vi "Main.vi"(8 "error in":errorcluster) -> (0 "error out":errorcluster)   [LabVIEW 2021, in "Interface-Module.lvlib"]
doc: "This template is based from the Queued Message Handler design pattern and the Queued Message Handler Project Template that ships with LabVIEW 2014.\n\nThe main difference is that the Queue is private to this module and communication between modules is done via Broadcast and Request events.\n\nRequest events are wrapped via public API methods and are handled in the Event handler loop in this VI.\nAny module can register for Broadcast events sent by this module.\n\nThe Event Handling Loop generates messages based on user interface actions.\n\nThe Message Handling Loop processes messages generated by the Event Handling Loop, or by other messages. The messages are string values, so new messages can be added easily to the Message Cases case structure in the Message Handling Loop. Each message cluster can also provide an optional value for Message Data, which is a variant that can be converted to whatever message-specific data is required.\n_____\nBased on Delacor QMH Project Template 3.0.0.32."
uses:
  Interface-Module.lvlib
  <vilib>/Delacor/Delacor QMH/Libraries/Module Admin_class/Delacor_lib_QMH_Module Admin.lvclass
  Module Data--cluster.ctl
  <vilib>/Delacor/Delacor QMH/Libraries/Message Queue_class/Delacor_lib_QMH_Message Queue.lvclass/Delacor_lib_QMH_Message Queue.ctl
  Valve-Module/Module/Controls/valve-cmd.ctl
  Show Panel Argument--cluster.ctl
  Hide Panel Argument--cluster.ctl
  Stop Argument--cluster.ctl
  <vilib>/Delacor/Delacor QMH/Libraries/Module Admin_class/Delacor_lib_QMH_Module Admin.lvclass/Delacor_lib_QMH_Module Admin.ctl
  <vilib>/Utility/miscctls.llb/LVPointTypeDef.ctl
  <vilib>/Delacor/Delacor QMH/Libraries/Message Queue_class/Delacor_lib_QMH_Enqueue Message (Single).vi
  <vilib>/Delacor/Delacor QMH/Libraries/Module Admin_class/Delacor_lib_QMH_Get External Launch.vi
  <vilib>/Utility/error.llb/Error Cluster From Error Code.vi
  <vilib>/ErrorRing/Error Ring.xnode
  <vilib>/Delacor/Delacor QMH/Libraries/Message Queue_class/Delacor_lib_QMH_Message Queue.lvclass
  Temperature-Module/Temperature-Module.lvlib
  Valve-Module/Valve-Module.lvlib
  Pressure Module/Pressure Module.lvlib
  Actuator Module/Actuator Module.lvlib
panel:
  out "Flow  2":dbl format="%_3g"
  out "Flow  1":dbl format="%_3g"
  out "P 5":dbl format="%_3g"
  out "P 4":dbl format="%_3g"
  out "P 3":dbl format="%_3g"
  out "P 2":dbl format="%_3g"
  out "P 1":dbl format="%_3g"
  out "Actuator Read":dbl(slide) scale=0.0..100.0
  out "Valve":bool[](array[boolean])
  out "Temperature":dbl[](array[numeric]) format="%#_4g"
  in  "Actuator\n Control":dbl(slide) scale=0.0..100.0
  in  "Start Display":bool
  in  "Valve 3":bool
  in  "Valve 2":bool
  in  "Valve 1":bool
  in  "Simulate MHL Error":bool
  in  "Simulate EHL Error":bool
  in  "Module Admin":refnum<class "Delacor_lib_QMH_Module Admin.lvclass">
  out "Status":string
  # "Distillation Column"
  # "Display"
  # "Control"
  # "Flow Meter"
  # "%"
  # "Pressure"
  # "Valve 1"
  # "Valve 2"
  # "Valve 3"
  # "Top"
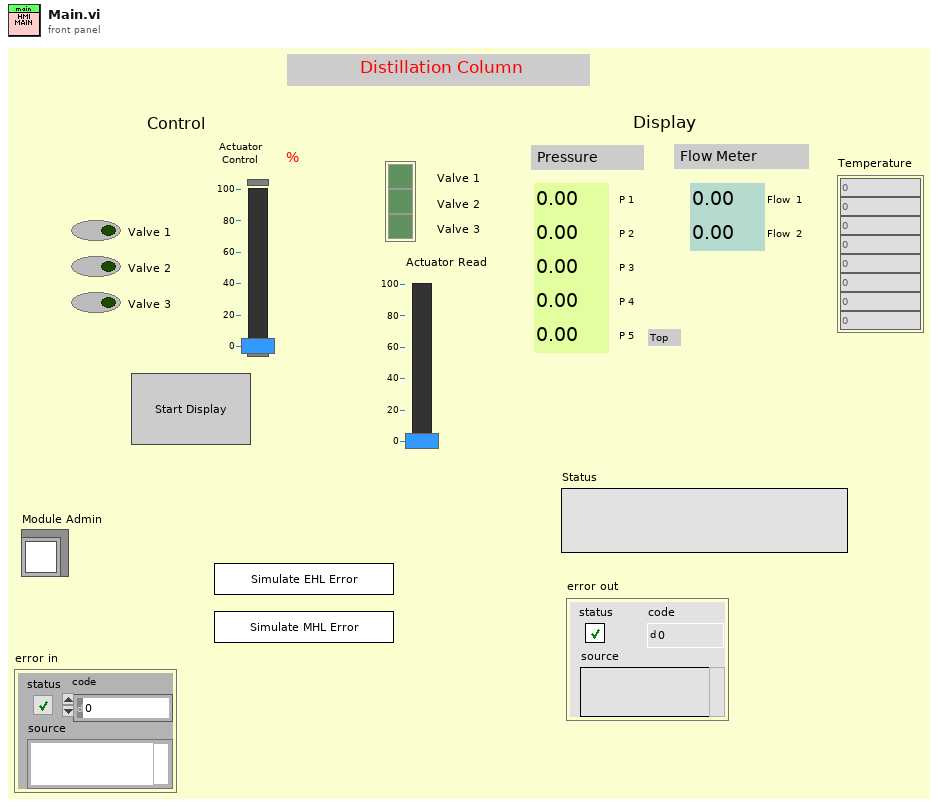
[diagram p1: front panel]
types:
  T1 = typedef "Interface-Module.lvlib/Request Events--cluster.ctl" = cluster{"Stop Module":refnum<user-event>, "Show Panel":refnum<user-event>, "Hide Panel":refnum<user-event>, "Get Module Execution Status":refnum<user-event>, "Show Diagram":refnum<user-event>}
  T2 = typedef "Temperature-Module.lvlib/Broadcast Events--cluster.ctl" = cluster{"Status Updated":refnum<user-event>, "Send Temperature to HMI":refnum<user-event>}
  T3 = typedef "Valve-Module.lvlib/Broadcast Events--cluster.ctl" = cluster{"Status Updated":refnum<user-event>, "Send-valve-interface":refnum<user-event>}
  T4 = typedef "Pressure Module.lvlib/Broadcast Events--cluster.ctl" = cluster{"Status Updated":refnum<user-event>, "Write pressure to HMI":refnum<user-event>}
  T5 = typedef "Actuator Module.lvlib/Broadcast Events--cluster.ctl" = cluster{"Status Updated":refnum<user-event>, "Actuator-display-Interface":refnum<user-event>}
  T6 = typedef "Interface-Module.lvlib/Module Data--cluster.ctl" = cluster{"Status":string}
  T7 = typedef "valve-cmd.ctl" = cluster{"Valve":bool, "Vavle Seq":i32}
  T8 = typedef "Interface-Module.lvlib/Show Panel Argument--cluster.ctl" = cluster{"Show Panel?":bool}
  T9 = typedef "Interface-Module.lvlib/Hide Panel Argument--cluster.ctl" = cluster{"Hide Panel?":bool}
  T10 = typedef "Interface-Module.lvlib/Stop Argument--cluster.ctl" = cluster{"Origin":string, "Exit via Stop Module Req?":bool, "Wait for Module to stop?":bool}
  T11 = typedef "LVPointTypeDef.ctl" = cluster{"Horizontal":i16, "Vertical":i16}
  T12 = enum32{"Invalid", "Standard", "Closed", "Hidden", "Minimized", "Maximized"}
  T13 = enum32{"invalid lock state", "Not Locked", "Locked (No Password)", "Password-protected"}
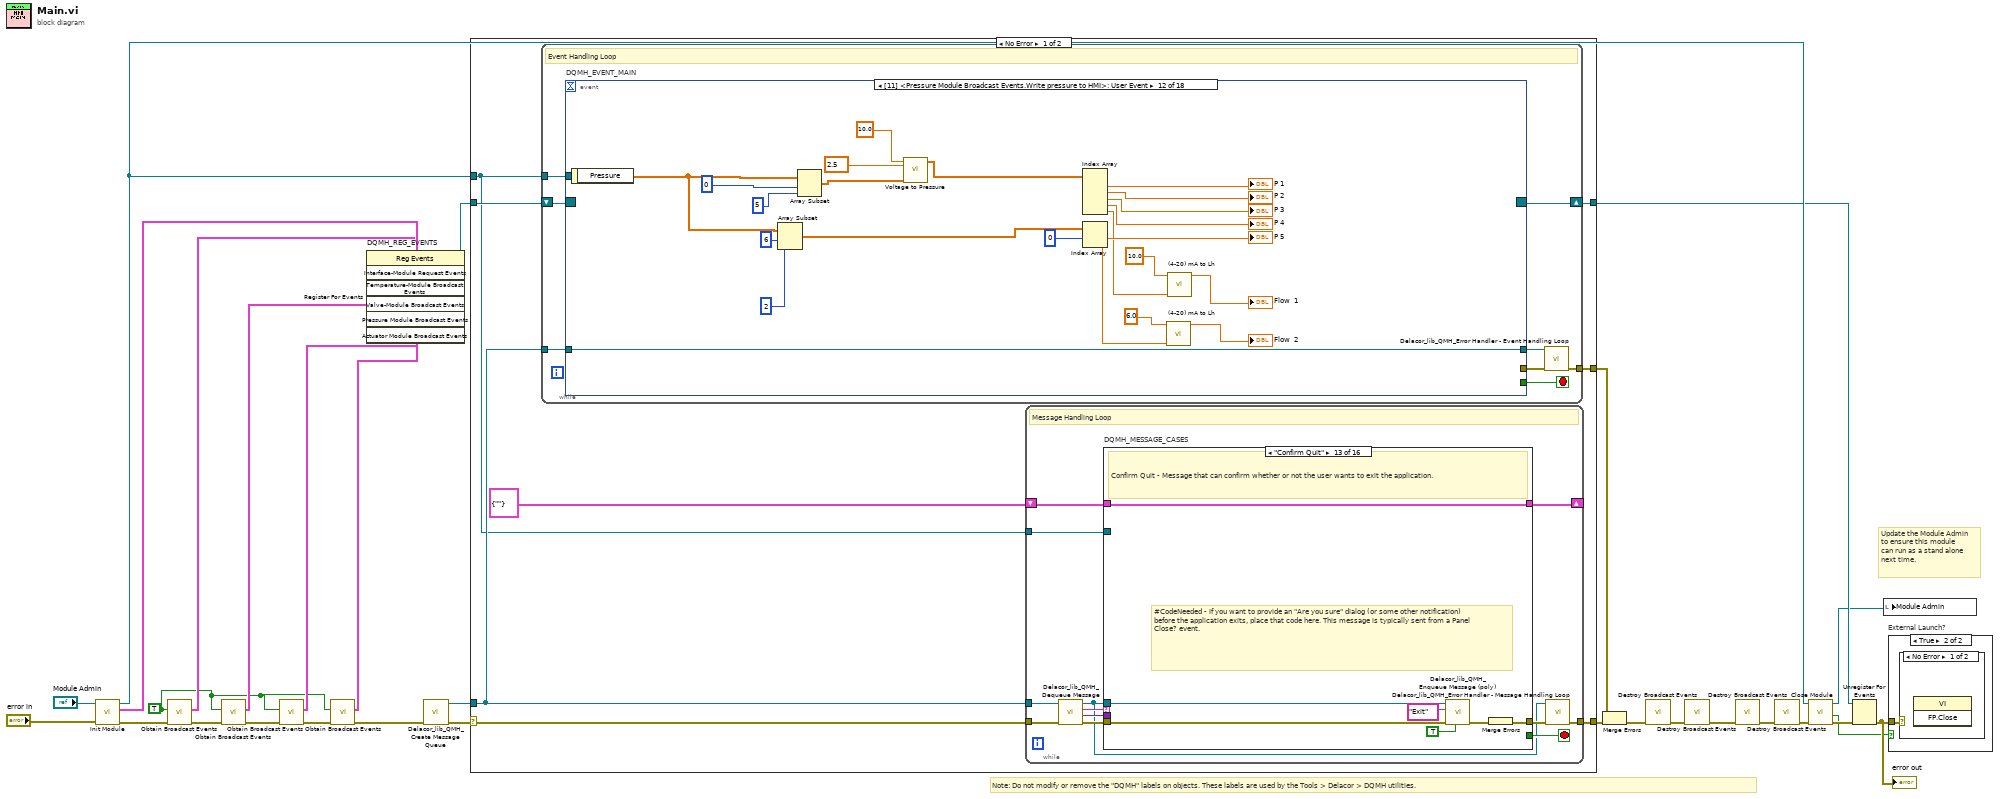
[diagram p0: block diagram]
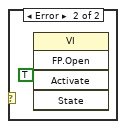
[diagram p3: hidden frame]
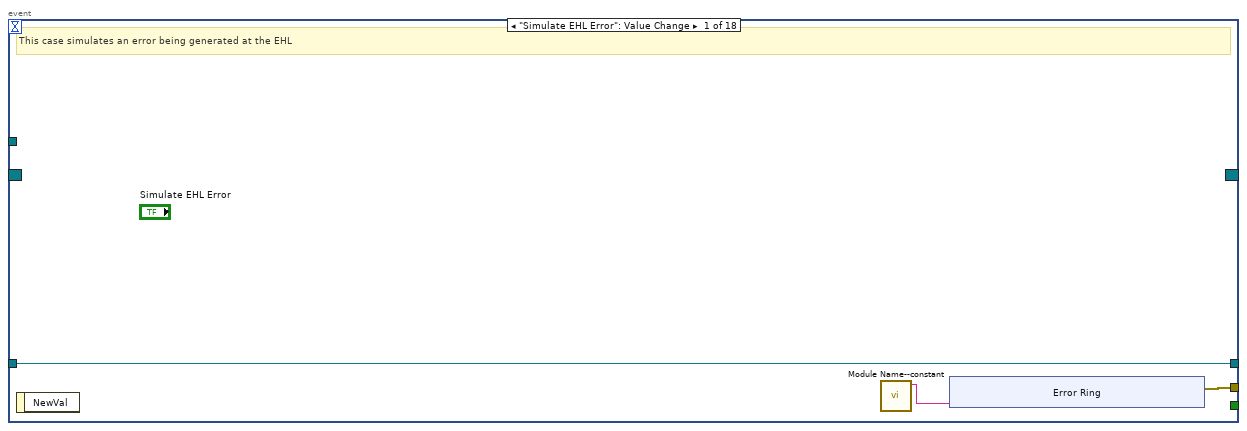
[diagram p4: hidden frame]
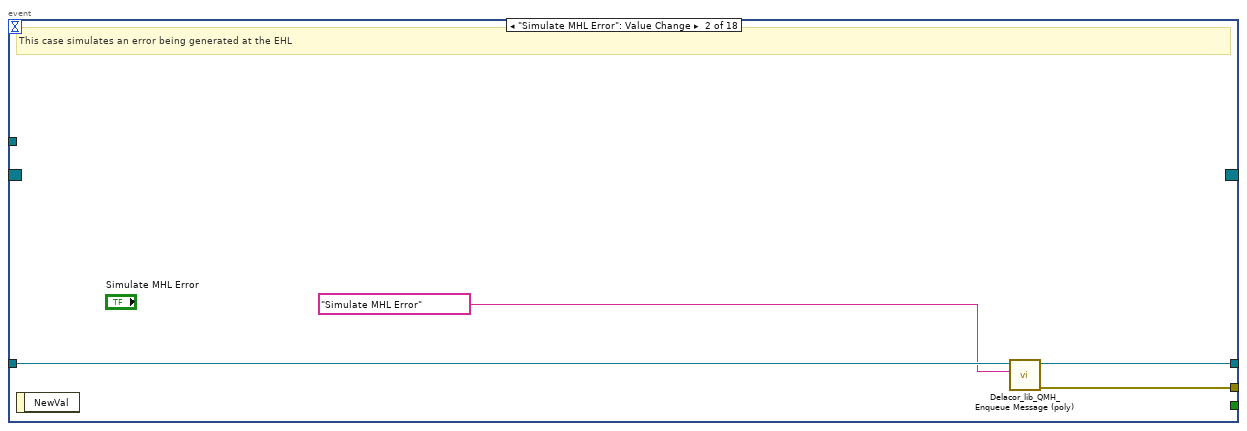
[diagram p5: hidden frame]
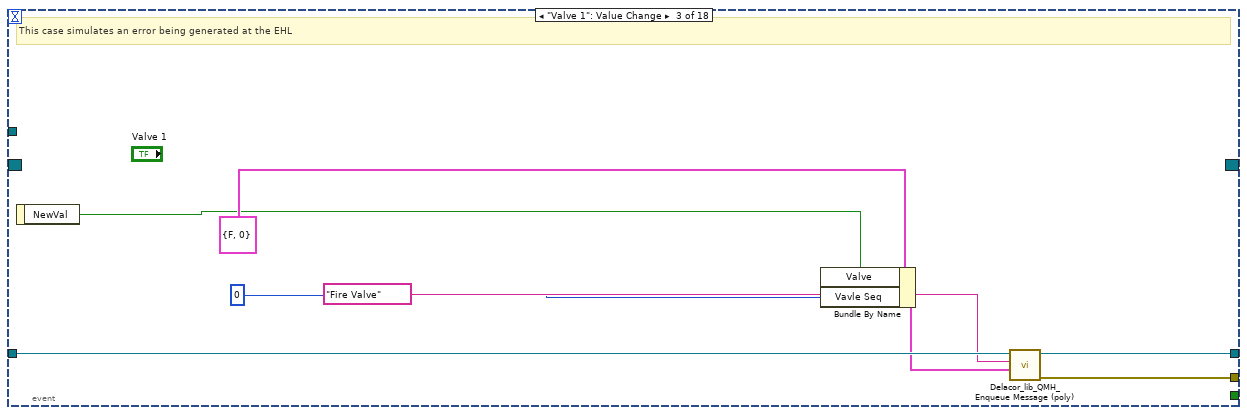
[diagram p6: hidden frame]
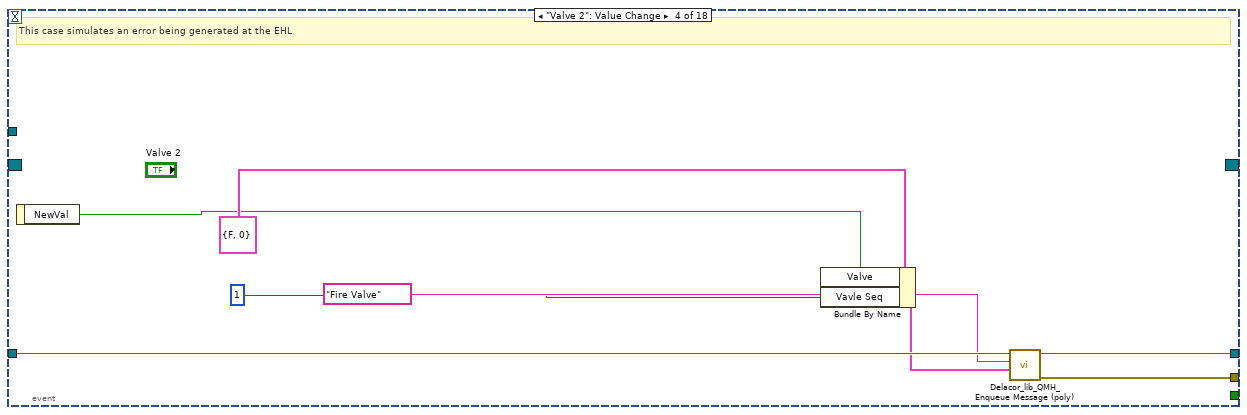
[diagram p7: hidden frame]
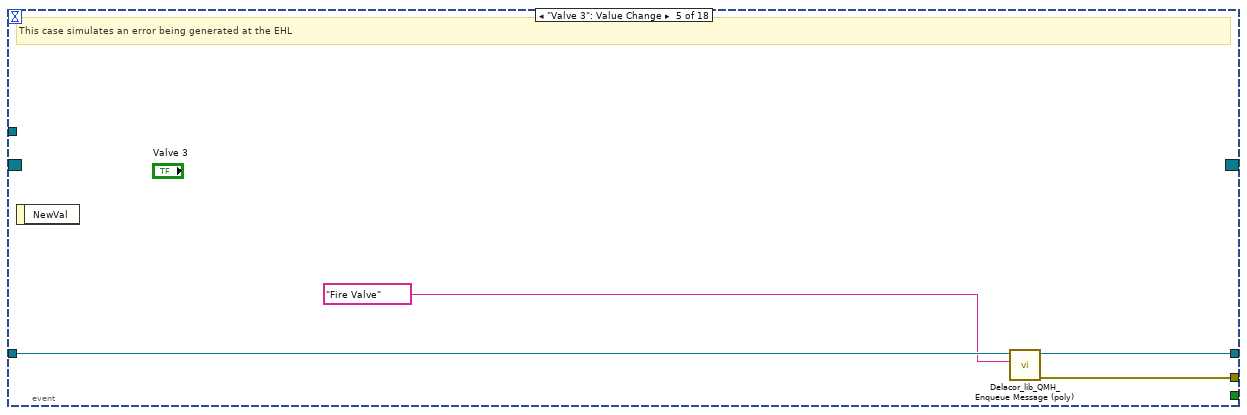
[diagram p8: hidden frame]
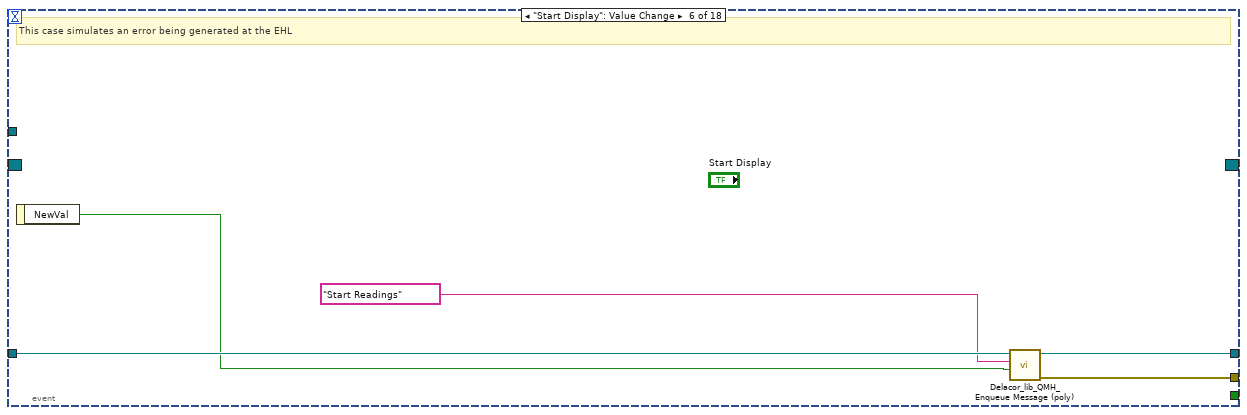
[diagram p9: hidden frame]
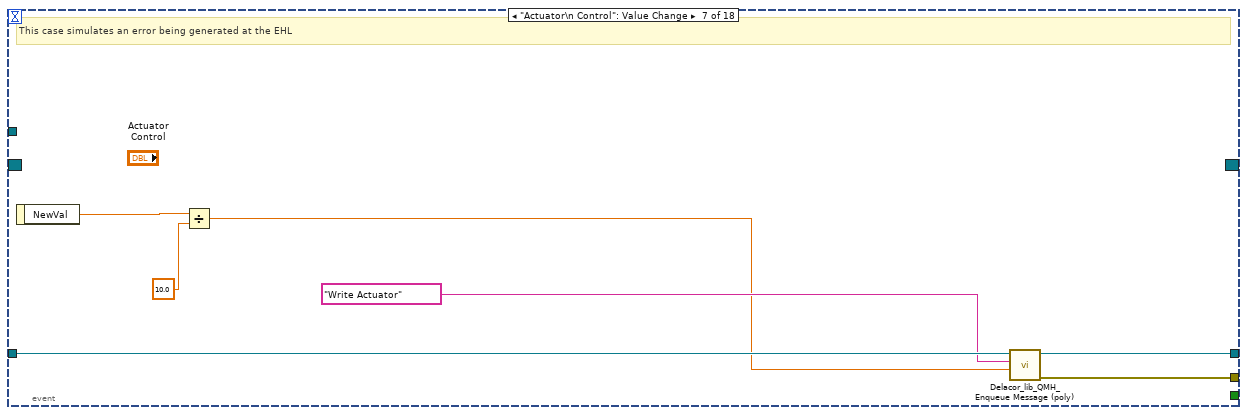
[diagram p10: hidden frame]
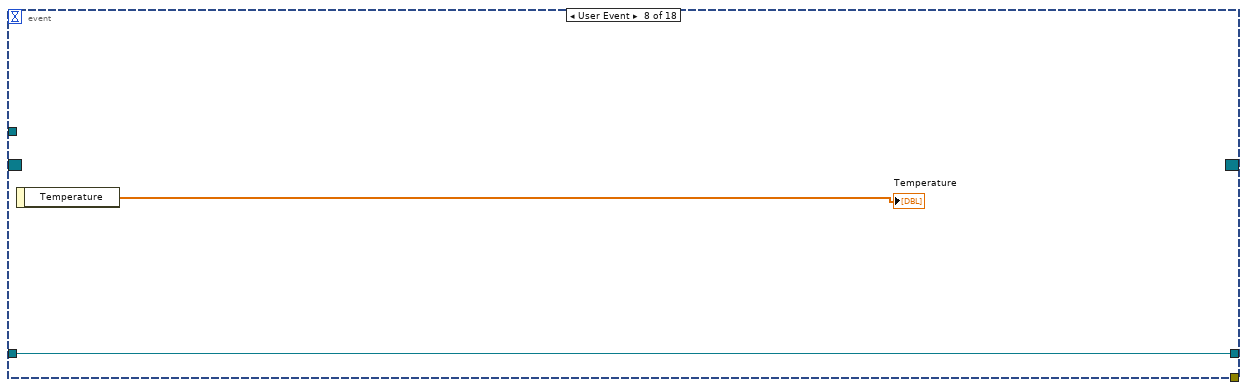
[diagram p11: hidden frame]
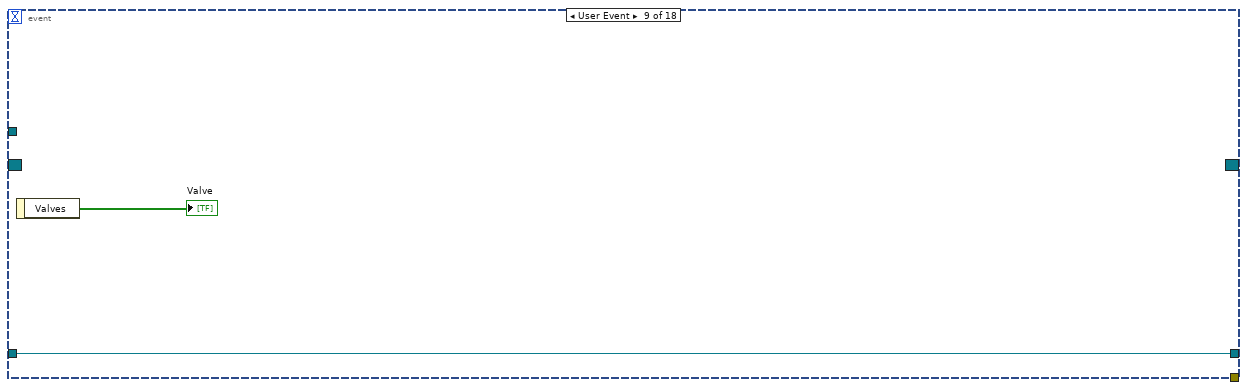
[diagram p12: hidden frame]
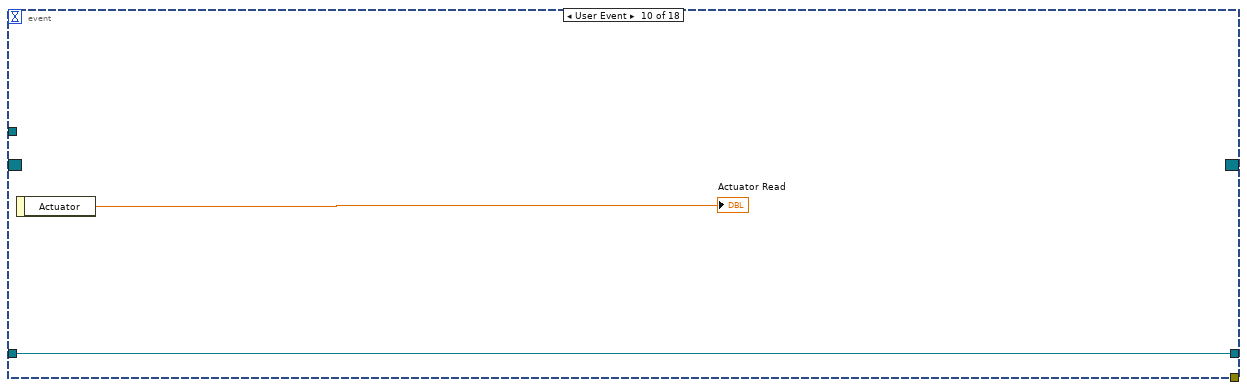
[diagram p13: hidden frame]
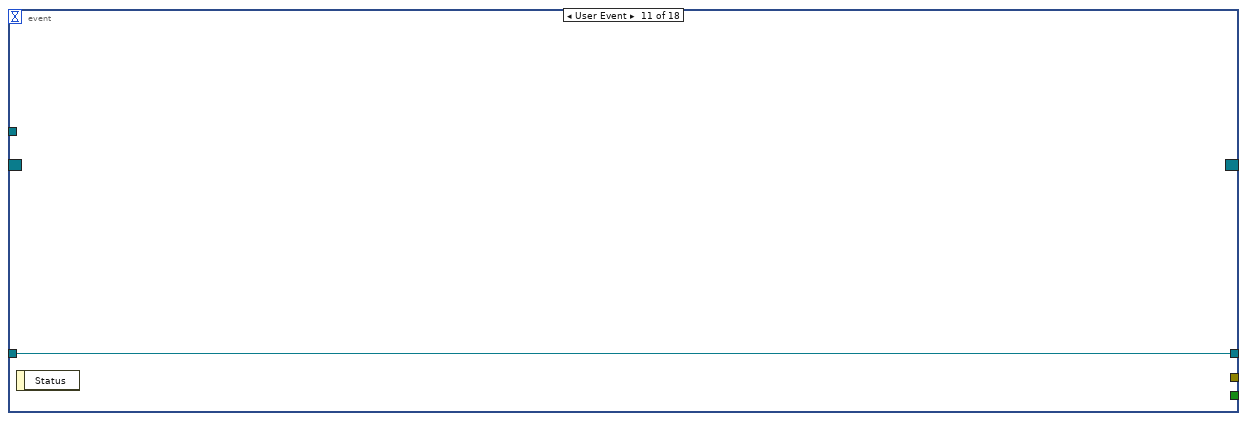
[diagram p14: hidden frame]
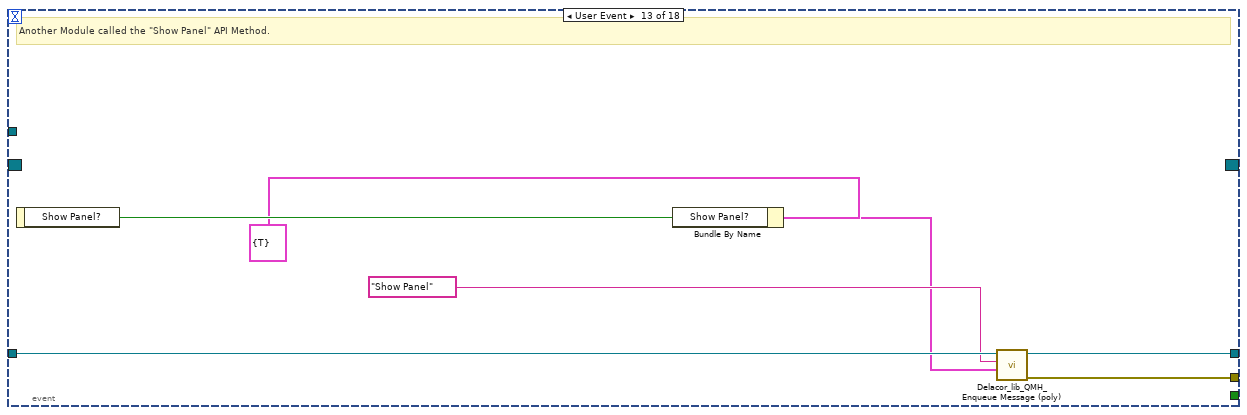
[diagram p15: hidden frame]
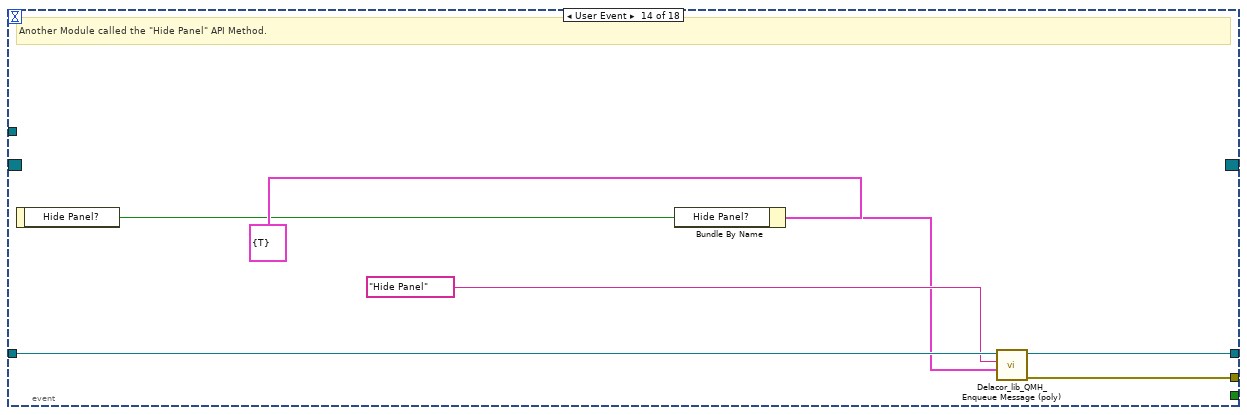
[diagram p16: hidden frame]
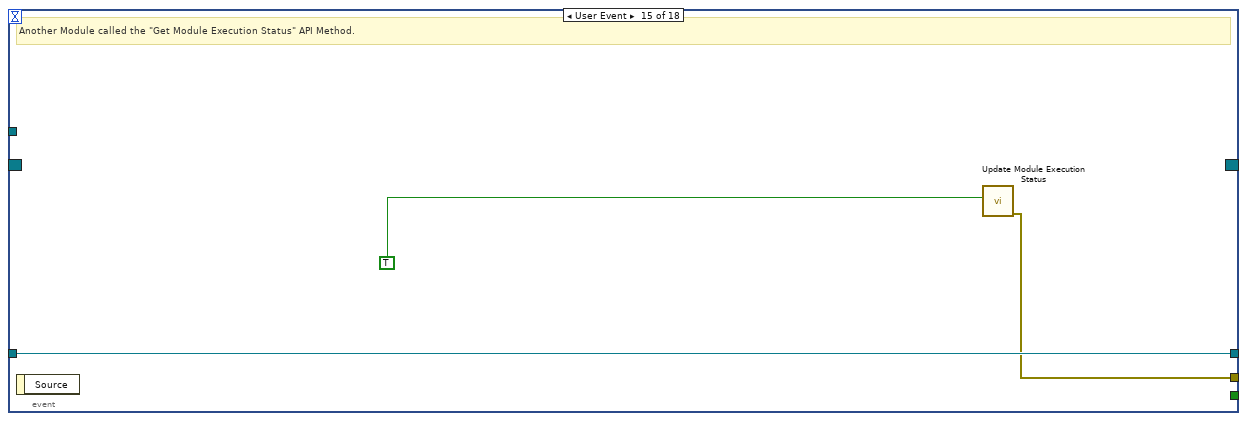
[diagram p17: hidden frame]
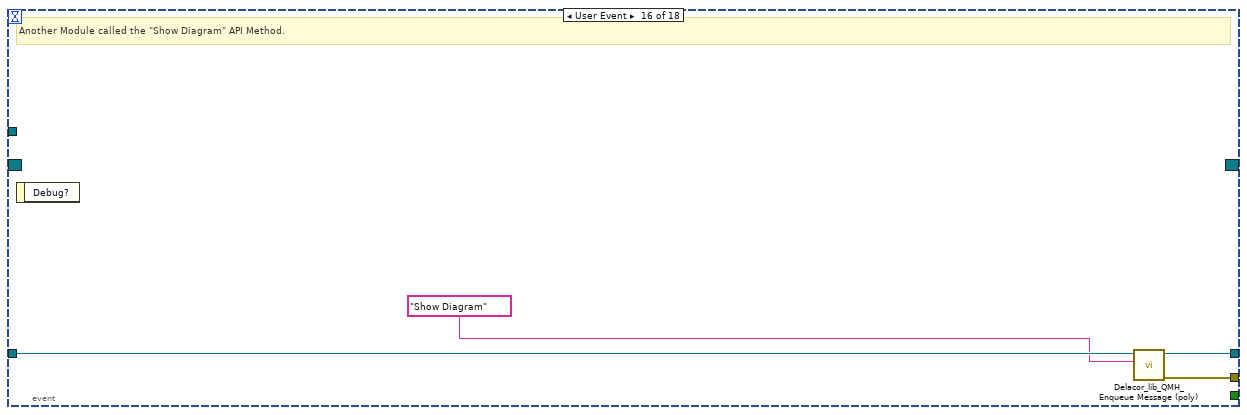
[diagram p18: hidden frame]
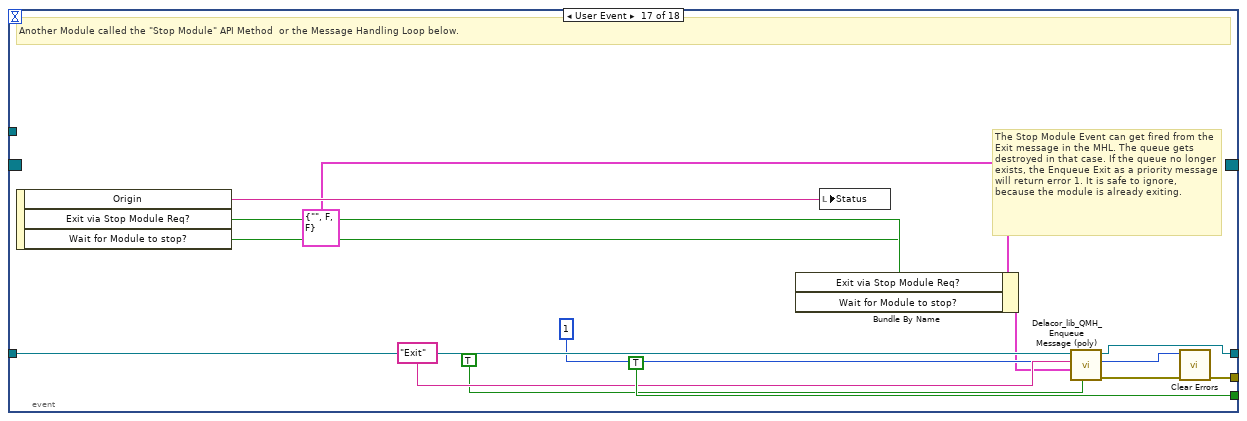
[diagram p19: hidden frame]
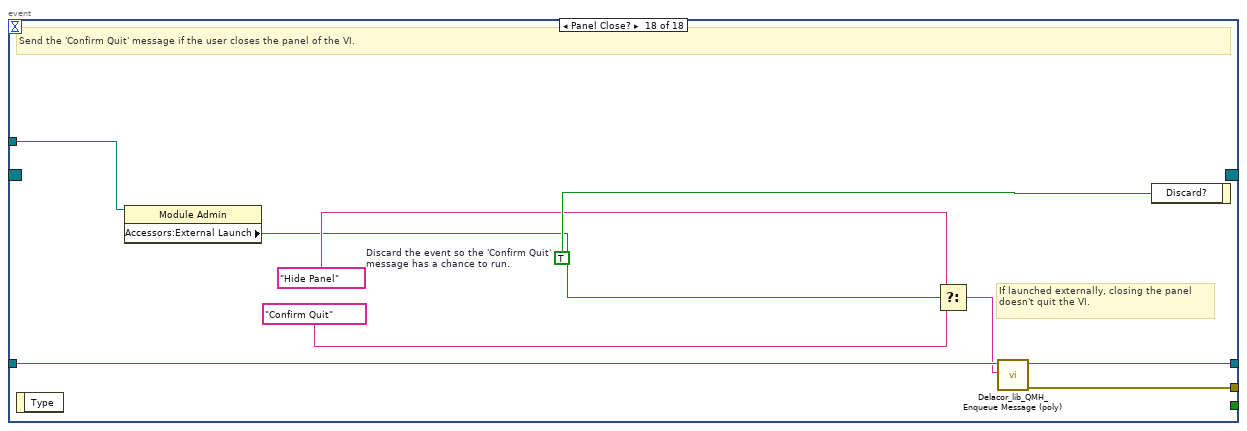
[diagram p20: hidden frame]
diagram:
  w4 = TRUE ("Create New?")
  # "Note: Do not modify or remove the \"DQMH\" labels on objects. These labels are used by the Tools > Delacor > DQMH utilities."
  # "Update the Module Admin to ensure this module can run as a stand alone next time."
  n1 = call "Init Module.vi"("error in (no error)"="error in", "Singleton Module Admin in"="Module Admin") -> ("error out"=w16:errorcluster, "Interface-Module Request Events"=w25:T1, "Singleton Module Admin out"=w29:refnum<class "Delacor_lib_QMH_Module Admin.lvclass">)  [unwired: 7 in]
  n2 = call "Obtain Broadcast Events.vi"("error in (no error)"=w16, "Create New?"=w4) -> ("error out"=w13:errorcluster, "Temperature-Module Broadcast Events"=w15:T2)  [unwired: 8 in]
  n3 = call "Obtain Broadcast Events.vi"("error in (no error)"=w13, "Create New?"=w4) -> ("error out"=w10:errorcluster, "Valve-Module Broadcast Events"=w12:T3)  [unwired: 8 in]
  n4 = call "Obtain Broadcast Events.vi"("error in (no error)"=w10, "Create New?"=w4) -> ("error out"=w6:errorcluster, "Pressure Module Broadcast Events"=w9:T4)  [unwired: 8 in]
  n5 = call "Obtain Broadcast Events.vi"("error in (no error)"=w6, "Create New?"=w4) -> ("error out"=w5:errorcluster, "Actuator Module Broadcast Events"=w3:T5)  [unwired: 8 in]
  n6 = register-events "DQMH_REG_EVENTS"(w25, w15, w12, w9, w3) -> (reference out=w26:refnum<event-registration>)  [unwired: 2 in, 1 out]
  n7 = call <vilib>:"Delacor_lib_QMH_Create Message Queue.vi"("error in"=w5) -> ("error out"=w17:errorcluster, "Message Queue"=w24:refnum<class "Delacor_lib_QMH_Message Queue.lvclass">)  [unwired: 9 in]
  n8 = case shown="No Error" w17 {
    selector: w17 -> [w31 w331]
    tunnel: [w37 w331] -> w28
    tunnel: [w36 w336] -> w27
    tunnel: w26 -> [w34 w336]
    tunnel: w24 -> [w33 _]
    tunnel: [w32 _] -> w20
    tunnel: w29 -> [w30 w332]
    frame No Error {
      n9 = while {
        tunnel: w33 -> [w45]
        shift-right: [w43] -> w36
        shift-left: w34 -> [w44]
        tunnel: [w39] -> w32
        tunnel: w30 -> [w38]
        stop <- w41 stop-if-true
        # "Event Handling Loop"
        n10 = event "DQMH_EVENT_MAIN" shown="[11] <Pressure Module Broadcast Events.Write pressure to HMI>: User Event" {
          selector: w44 -> [_ _ _ _ _ _ _ _ _ _ _ _ _ _ _ _ _ _]
          dyn-events: [_ _ _ _ _ _ _ _ _ _ _ _ _ _ _ _ _ _] -> w43
          timeout: _ -> [_ _ _ _ _ _ _ _ _ _ _ _ _ _ _ _ _ _]
          tunnel: [_ _ _ _ _ _ _ _ _ _ _ _ _ _ _ _ TRUE ("Discard?") _] -> w41
          tunnel: w45 -> [w48 w59 w67 w75 w79 w84 w91 w93 w95 w97 w98 w121 w128 w135 w138 w142 w153 w163]
          tunnel: [w47 w56 w64 w72 w76 w81 w88 _ _ _ _ _ w126 w133 w137 w139 w147 w162] -> w42
          tunnel: [w48 w58 w66 w74 w78 w83 w90 w93 w95 w97 w98 w121 w127 w134 w138 w141 w152 w161] -> w40
          tunnel: w38 -> [_ _ _ _ _ _ _ _ _ _ _ _ _ _ _ _ _ w157]
          event "Simulate EHL Error": Value Change {
            # "This case simulates an error being generated at the EHL"
            n11 = event-data() -> ()  [unwired: 1 in, 1 out]
            n12 = call "Module Name--constant.vi"() -> ("Module Name"=w46:string)  [unwired: 11 in]
            n13 = xnode "Error Ring"("parameter 0"=w46) -> ("error out"=w47:errorcluster)
          }
          event "Simulate MHL Error": Value Change {
            # "This case simulates an error being generated at the EHL"
            n14 = event-data() -> ()  [unwired: 1 in, 1 out]
            n15 = call-poly <vilib>:"Delacor_lib_QMH_Enqueue Message (poly).vi"("Message"="Simulate MHL Error", "Message Queue in"=w59) -> ("error out"=w56:errorcluster, "Message Queue out"=w58:refnum<class "Delacor_lib_QMH_Message Queue.lvclass">)  [unwired: 8 in]
          }
          event "Valve 1": Value Change {
            # "This case simulates an error being generated at the EHL"
            n16 = event-data() -> ("NewVal"=w62:bool)  [unwired: 1 in]
            n17 = Bundle By Name(cluster=T7 {"Valve"=FALSE, "Vavle Seq"=0} ("Cmd"), "Valve"=w62, "Vavle Seq"=0) -> (w60:T7)
            n18 = call-poly <vilib>:"Delacor_lib_QMH_Enqueue Message (poly).vi"("Message Data"=w60, "Message"="Fire Valve", "Message Queue in"=w67) -> ("error out"=w64:errorcluster, "Message Queue out"=w66:refnum<class "Delacor_lib_QMH_Message Queue.lvclass">)  [unwired: 7 in]
          }
          event "Valve 2": Value Change {
            # "This case simulates an error being generated at the EHL"
            n19 = event-data() -> ("NewVal"=w70:bool)  [unwired: 1 in]
            n20 = Bundle By Name(cluster=T7 {"Valve"=FALSE, "Vavle Seq"=0} ("Cmd"), "Valve"=w70, "Vavle Seq"=1) -> (w68:T7)
            n21 = call-poly <vilib>:"Delacor_lib_QMH_Enqueue Message (poly).vi"("Message Data"=w68, "Message"="Fire Valve", "Message Queue in"=w75) -> ("error out"=w72:errorcluster, "Message Queue out"=w74:refnum<class "Delacor_lib_QMH_Message Queue.lvclass">)  [unwired: 7 in]
          }
          event "Valve 3": Value Change {
            # "This case simulates an error being generated at the EHL"
            n22 = event-data() -> ()  [unwired: 1 in, 1 out]
            n23 = call-poly <vilib>:"Delacor_lib_QMH_Enqueue Message (poly).vi"("Message"="Fire Valve", "Message Queue in"=w79) -> ("error out"=w76:errorcluster, "Message Queue out"=w78:refnum<class "Delacor_lib_QMH_Message Queue.lvclass">)  [unwired: 8 in]
          }
          event "Start Display": Value Change {
            # "This case simulates an error being generated at the EHL"
            n24 = event-data() -> ("NewVal"=w80:bool)  [unwired: 1 in]
            n25 = call-poly <vilib>:"Delacor_lib_QMH_Enqueue Message (poly).vi"("Message Data"=w80, "Message"="Start Readings", "Message Queue in"=w84) -> ("error out"=w81:errorcluster, "Message Queue out"=w83:refnum<class "Delacor_lib_QMH_Message Queue.lvclass">)  [unwired: 7 in]
          }
          event "Actuator\n Control": Value Change {
            # "This case simulates an error being generated at the EHL"
            n26 = event-data() -> ("NewVal"=w87:dbl)  [unwired: 1 in]
            n27 = Divide(x=w87, y=10.0) -> (x/y=w86:dbl)
            n28 = call-poly <vilib>:"Delacor_lib_QMH_Enqueue Message (poly).vi"("Message Data"=w86, "Message"="Write Actuator", "Message Queue in"=w91) -> ("error out"=w88:errorcluster, "Message Queue out"=w90:refnum<class "Delacor_lib_QMH_Message Queue.lvclass">)  [unwired: 7 in]
          }
          event User Event {
            n29 = event-data() -> ("Temperature"=→"Temperature":dbl[])  [unwired: 1 in]
          }
          event User Event {
            n30 = event-data() -> ("Valves"=→"Valve":bool[])  [unwired: 1 in]
          }
          event User Event {
            n31 = event-data() -> ("Actuator"=→"Actuator Read":dbl)  [unwired: 1 in]
          }
          event User Event {
            n32 = event-data() -> ()  [unwired: 1 in, 1 out]
          }
          event User Event {
            n33 = event-data() -> ("Pressure"=w114:dbl[])  [unwired: 1 in]
            n34 = Array Subset(array=w114, index=6, length=2) -> (w116:dbl[])
            n35 = Array Subset(array=w114, index=0, length=5) -> (w111:dbl[])
            n36 = call "Voltage to Pressure.vi"("x"=w111, "Vmax"=2.5, "Pmax"=10.0) -> ("pressureOut"=w110:dbl[])  [unwired: 8 in]
            n37 = Index Array "Index Array"(array=w110) -> (element #1=→"P 1":dbl, element #2=→"P 2":dbl, element #3=→"P 3":dbl, element #4=→"P 4":dbl, element #5=→"P 5":dbl)  [unwired: 5 in]
            n38 = Index Array "Index Array"(array=w116, index #1=0 ("index")) -> (element #1=w104:dbl, element #2=w101:dbl)  [unwired: 1 in]
            n39 = call "(4-20) mA to Lh.vi"("x"=w101, "flowMax"=6.0) -> ("flowOut"=→"Flow  2":dbl)  [unwired: 9 in]
            n40 = call "(4-20) mA to Lh.vi"("x"=w104, "flowMax"=10.0) -> ("flowOut"=→"Flow  1":dbl)  [unwired: 9 in]
          }
          event User Event {
            # "Another Module called the \"Show Panel\" API Method."
            n41 = event-data() -> ("Show Panel?"=w124:bool)  [unwired: 1 in]
            n42 = Bundle By Name(cluster=T8 {"Show Panel?"=TRUE} ("Show Panel Argument"), "Show Panel?"=w124) -> (w122:T8)
            n43 = call-poly <vilib>:"Delacor_lib_QMH_Enqueue Message (poly).vi"("Message Data"=w122, "Message"="Show Panel", "Message Queue in"=w128) -> ("error out"=w126:errorcluster, "Message Queue out"=w127:refnum<class "Delacor_lib_QMH_Message Queue.lvclass">)  [unwired: 7 in]
          }
          event User Event {
            # "Another Module called the \"Hide Panel\" API Method."
            n44 = event-data() -> ("Hide Panel?"=w130:bool)  [unwired: 1 in]
            n45 = Bundle By Name(cluster=T9 {"Hide Panel?"=TRUE} ("Hide Panel Argument"), "Hide Panel?"=w130) -> (w129:T9)
            n46 = call-poly <vilib>:"Delacor_lib_QMH_Enqueue Message (poly).vi"("Message Data"=w129, "Message"="Hide Panel", "Message Queue in"=w135) -> ("error out"=w133:errorcluster, "Message Queue out"=w134:refnum<class "Delacor_lib_QMH_Message Queue.lvclass">)  [unwired: 7 in]
          }
          event User Event {
            # "Another Module called the \"Get Module Execution Status\" API Method."
            n47 = event-data() -> ()  [unwired: 1 in, 1 out]
            n48 = call "Update Module Execution Status.vi"("Running?"=TRUE) -> ("error out"=w137:errorcluster)  [unwired: 10 in]
          }
          event User Event {
            # "Another Module called the \"Show Diagram\" API Method."
            n49 = event-data() -> ()  [unwired: 1 in, 1 out]
            n50 = call-poly <vilib>:"Delacor_lib_QMH_Enqueue Message (poly).vi"("Message"="Show Diagram", "Message Queue in"=w142) -> ("error out"=w139:errorcluster, "Message Queue out"=w141:refnum<class "Delacor_lib_QMH_Message Queue.lvclass">)  [unwired: 8 in]
          }
          event User Event {
            # "The Stop Module Event can get fired from the Exit message in the MHL. The queue gets destroyed in that case. If the queue no longer exists, the Enqueue Exit as a priority message will return error 1. It is safe to ignore, because the module is already exiting."
            # "Another Module called the \"Stop Module\" API Method  or the Message Handling Loop below."
            n51 = event-data() -> ("Origin"=w151:string, "Exit via Stop Module Req?"=w145:bool, "Wait for Module to stop?"=w144:bool)  [unwired: 1 in]
            n52 = Bundle By Name(cluster=T10 {"Origin"="", "Exit via Stop Module Req?"=FALSE, "Wait for Module to stop?"=FALSE} ("Stop Argument"), "Exit via Stop Module Req?"=w145, "Wait for Module to stop?"=w144) -> (w143:T10)
            n53 = local write "Status"(w151) -> ()
            n54 = call-poly <vilib>:"Delacor_lib_QMH_Enqueue Message (poly).vi"("Priority Message? (F)"=TRUE, "Message Data"=w143, "Message"="Exit", "Message Queue in"=w153) -> ("error out"=w148:errorcluster, "Message Queue out"=w152:refnum<class "Delacor_lib_QMH_Message Queue.lvclass">)  [unwired: 6 in]
            n55 = call <vilib>:"Clear Errors.vi"("error in (no error)"=w148, "specific error code to clear (0: all)"=1) -> ("error out"=w147:errorcluster)  [unwired: 4 in, 1 out]
          }
          event Panel Close? {
            w164 = TRUE  # Discard the event so the 'Confirm Quit' message has a chance to run.
            # "If launched externally, closing the panel doesn't quit the VI."
            # "Send the 'Confirm Quit' message if the user closes the panel of the VI."
            n56 = event-data() -> ()  [unwired: 1 in, 1 out]
            n57 = property class="Module Admin"(reference=w157) -> ("Accessors:External Launch"=w156:bool)  [unwired: 1 in, 2 out]
            n58 = Select(t="Hide Panel" ("Message"), s=w156, f="Confirm Quit" ("Message")) -> (s? t:f=w158:string)
            n59 = call-poly <vilib>:"Delacor_lib_QMH_Enqueue Message (poly).vi"("Message"=w158, "Message Queue in"=w163) -> ("error out"=w162:errorcluster, "Message Queue out"=w161:refnum<class "Delacor_lib_QMH_Message Queue.lvclass">)  [unwired: 8 in]
            n60 = event-data("Discard?"=w164) -> ()  [unwired: 1 in, 1 out]
          }
        }
        n61 = call-dynamic "Delacor_lib_QMH_Error Handler - Event Handling Loop.vi"("error in"=w42, "Message Queue in"=w40) -> ("dup error in"=w39:errorcluster)  [unwired: 8 in, 1 out]
      }
      n62 = while {
        tunnel: w33 -> [w168]
        shift-right: [w174] -> _
        shift-left: T6 {"Status"=""} ("Data Cluster") -> [w175]
        tunnel: w31 -> [w172]
        tunnel: [w166] -> w37
        tunnel: w30 -> [w165]
        stop <- w173 stop-if-true
        # "Message Handling Loop"
        n63 = call-dynamic "Delacor_lib_QMH_Dequeue Message.vi"("error in"=w172, "Message Queue in"=w168) -> ("error out"=w171:errorcluster, "Message Data"=w169:variant, "Message"=w170:string, "Message Queue out"=w167:refnum<class "Delacor_lib_QMH_Message Queue.lvclass">)  [unwired: 6 in]
        n64 = case "DQMH_MESSAGE_CASES" shown="\"Confirm Quit\"" w170 {
          selector: w170 -> [_ _ _ _ _ _ _ _ _ _ _ _ _ _ _ w318]
          tunnel: w167 -> [_ _ _ _ _ _ _ _ _ _ _ w270 w285 w307 _ _]
          tunnel: w171 -> [w186 w202 w211 w218 w224 w225 w230 w248 w251 w254 w259 w276 w289 w309 w316 _]
          tunnel: [w179 w203 w212 w219 w224 w225 w229 w246 w249 w252 w257 w267 w287 w303 w314 w319] -> w176
          tunnel: w175 -> [w185 w204 w213 w220 w223 w228 w231 w247 w250 w253 w258 w275 w288 w306 w315 w320]
          tunnel: [w184 w204 w213 w220 w223 w228 w231 w247 w250 w253 w258 w275 w288 w306 w315 w320] -> w174
          tunnel: [_ _ _ _ _ _ _ _ _ _ _ _ _ w305 _ _] -> w173
          tunnel: w169 -> [_ w201 _ w216 _ _ _ _ _ _ _ w274 _ w302 w313 _]
          tunnel: w165 -> [w187 _ _ _ _ _ _ _ _ _ _ w269 _ w295 _ _]
          frame "Initialize" {
            w183 = "Initial Message" ("Initial Message")
            # "#CodeNeeded - Initialize the appearance of the front panel."
            # "#CodeNeeded - Initialize your state data here."
            # "Initialize - Any operation that needs to be done before the module can receive messages. Synchronize Caller Events.vi will inform Start Module.vi that the module has launched and is ready to receive messages. Module Did Init.vi will broadcast that the module initialized."
            n65 = call "Synchronize Caller Events.vi"("error in (no error)"=w186, "Singleton Module Admin in"=w187) -> ("error out"=w180:errorcluster, "Singleton Module Admin out"=w178:refnum<class "Delacor_lib_QMH_Module Admin.lvclass">)  [unwired: 8 in]
            n66 = property class="Module Admin"(reference=w178) -> ("Accessors:External Launch"=w191:bool)  [unwired: 1 in, 2 out]
            n67 = Select(t=T12."Hidden" ("State"), s=w191, f=T12."Standard" ("State")) -> (s? t:f=w188:T12)
            n68 = call "Module Name--constant.vi"() -> ("Module Name"=w196:string)  [unwired: 11 in]
            n69 = property class="VI"("Front Panel.Title"=w196) -> (reference out=w194:refnum<vi>, error out=w195:errorcluster)  [unwired: 2 in]
            n70 = call "Module Name--constant.vi"() -> ("Module Name"=w181:string)  [unwired: 11 in]
            n71 = invoke class="VI" method="FP.Open"(reference=w194, error in=w195, "State"=w188) -> (reference out=w193:refnum<vi>, error out=w192:errorcluster)  [unwired: 2 in, 3 out]
            n72 = Bundle By Name(cluster=w185, "Status"=w183) -> (w184:T6)
            n73 = local write "Status"(w183) -> ()
            n74 = call "Module Did Init.vi"("error in (no error)"=w180, "Initialized?"=TRUE, "Origin"=w181) -> ("error out"=w179:errorcluster)  [unwired: 8 in]
            n75 = invoke class="VI" method="FP.Center"(reference=w193, error in=w192) -> ()  [unwired: 1 in, 3 out]
            n76 = property on="Pane" class="Pane"("Origin"=T11 {"Horizontal"=0, "Vertical"=0}) -> ()  [unwired: 2 in, 2 out]
          }
          frame "Update Display" {
            # "Broadcast updated status to any VI registered to listen to this module's broadcast events."
            # "Convert the message data to a string to display in the Status indicator."
            # "#CodeRecommended - If you wish to decouple the Message Handling Loop from your user interface, consider creating User Events (like the \"Stop\" event in this VI) to message the Event Handling Loop whenever the user interface needs updating."
            # "Update Display - Update user interface here."
            n77 = Variant To Data(error in=w202, type="", Variant=w201) -> (data=w199:string, error out=w198:errorcluster)
            "Status" <- w199
            n78 = call "Status Updated.vi"("error in (no error)"=w198, "Status"=w199) -> ("error out"=w197:errorcluster)  [unwired: 9 in]
            n79 = Merge Errors(w197) -> (w203:errorcluster)
          }
          frame "Fire Valve" {
            # "Update Display - Update user interface here."
            n80 = local read "Valve 1"() -> (w206:bool)
            n81 = local read "Valve 2"() -> (w207:bool)
            n82 = local read "Valve 3"() -> (w208:bool)
            n83 = Insert Into Array(array=bool[] [FALSE], index=0, new element #1=w206, new element #2=w207, new element #3=w208) -> (w205:bool[])
            n84 = call "Write Fire Valves.vi"("Valves"=w205) -> ()  [unwired: 10 in, 1 out]
            n85 = Merge Errors(w211) -> (w212:errorcluster)
          }
          frame "Start Readings" {
            # "Update Display - Update user interface here."
            n86 = Variant To Data(error in=w218, type=FALSE, Variant=w216) -> (data=w214:bool, error out=w217:errorcluster)
            n87 = call "Start Temp Display.vi"("Temperature"=w214) -> ()  [unwired: 10 in, 1 out]
            n88 = call "Start Display Pressure.vi"("Pressure"=w214) -> ()  [unwired: 10 in, 1 out]
            n89 = Merge Errors(w217) -> (w219:errorcluster)
          }
          frame "Show Panel" {
            # "Show the panel of this VI, and send a status updated message to let listeners know."
            n90 = call "Status Updated.vi"("Status"="Panel shown." ("format string")) -> ()  [unwired: 10 in, 1 out]
            n91 = invoke class="VI" method="FP.Open"("Activate"=TRUE ("Activate?")) -> ()  [unwired: 4 in, 5 out]
          }
          frame "Hide Panel" {
            # "Hide the panel of this VI, and send a status updated message to let listeners know."
            n92 = call "Status Updated.vi"("Status"="Panel hidden." ("format string")) -> ()  [unwired: 10 in, 1 out]
            n93 = invoke class="VI" method="FP.Open"("State"=T12."Hidden") -> ()  [unwired: 4 in, 5 out]
          }
          frame "Show Diagram" {
            # "Show Diagram - Show the block diagram of this VI. Used as a debugging tool. There is a button in the module tester that fires the Show Diagram request, which runs this message. Note that the diagram will not be displayed if it is password-protected and the password is not in the cache."
            n94 = disable-structure shown="Default" {
              disable-tunnel: [w239 w245] -> w229
              disable-tunnel: w230 -> [w238 w245]
              frame condition #0 (active) {
                # "functionality not available in exe"
                n95 = invoke class="VI" method="Lock State.Get"(error in=w238) -> (error out=w237:errorcluster, "Get Lock State"=w236:T13, "pwd in cache"=w233:bool)  [unwired: 3 in, 1 out]
                n96 = Equal?(x=T13."Password-protected", y=w236) -> (x = y?=w234:bool)
                n97 = Compound Arithmetic op=AND(w234, invert w233) -> (w232:bool)
                n98 = case shown="False" w232 {
                  tunnel: [w242 w244] -> w239
                  tunnel: w237 -> [w240 w244]
                  frame False {
                    n99 = property class="VI"(error in=w240, "BDWin.Open"=TRUE ("Block Diagram Window:Open")) -> (error out=w242:errorcluster)  [unwired: 1 in, 1 out]
                    n100 = call "Status Updated.vi"("Status"="Block Diagram shown." ("format string")) -> ()  [unwired: 10 in, 1 out]
                  }
                  frame True {
                    # "Password-protected VI, and the password is not in the cache. Do not show the diagram."
                  }
                }
              }
              frame condition #1 {
              }
            }
          }
          frame "--- Module Specific ---" {
            # "Separator -- The following cases handle messages specific to this Module."
            n101 = Merge Errors(w248) -> (w246:errorcluster)
          }
          frame "---Copy This Frame---" {
            # "Duplicate this frame when creating new messages.  Change this comment in the duplicated frame to describe this message."
            n102 = Merge Errors(w251) -> (w249:errorcluster)
          }
          frame "--- Exit and Error Handling---" {
            # "Separator - The following cases handle errors and exit messages."
            n103 = Merge Errors(w254) -> (w252:errorcluster)
          }
          frame "Simulate MHL Error" {
            # "Simulate an error occurring at the MHL"
            n104 = call "Module Name--constant.vi"() -> ("Module Name"=w256:string)  [unwired: 11 in]
            n105 = xnode "Error Ring"("parameter 0"=w256) -> ("error out"=w255:errorcluster)
            n106 = Merge Errors(w259, w255) -> (w257:errorcluster)
          }
          frame "Error" {
            # "#CodeRecommended - If you ever change the name of this \"Error\" message, you'll need to update the name in the Check Loop Error.vi as well."
            # "#CodeRecommended - If the module is running in standalone mode (External Launch = FALSE), this code will pop up an error dialog and call the 'Exit' message if an error occurs. Add more fine-grained error handling here."
            # "Error - Check the error message data and respond accordingly. This message is sent by the \"Error Handler\" VIs at the end of each loop in this application."
            n107 = property class="Module Admin"(reference=w269) -> ("Accessors:External Launch"=w268:bool)  [unwired: 1 in, 2 out]
            n108 = Variant To Data(error in=w276, type=errorcluster {"status"=FALSE, "code"=0, "source"=""} ("error constant"), Variant=w274) -> (data=w277:errorcluster, error out=w272:errorcluster)
            n109 = call "Error Reported.vi"("Error"=w277) -> ()  [unwired: 10 in, 1 out]
            n110 = case shown="False" w268 {
              tunnel: [w282 _] -> w271
              tunnel: w270 -> [w281 _]
              tunnel: w277 -> [w278 _]
              frame False {
                # "If the module is running standalone, then pop up an error dialog and call the \"Exit\" message."
                n111 = call <vilib>:"Simple Error Handler.vi"("error in (no error)"=w278) -> ()  [unwired: 4 in, 5 out]
                n112 = call-poly <vilib>:"Delacor_lib_QMH_Enqueue Message (poly).vi"("Priority Message? (F)"=TRUE, "Message"="Exit", "Message Queue in"=w281) -> ("error out"=w282:errorcluster)  [unwired: 7 in, 1 out]
              }
              frame True {
                # "If the module was launched externally, calling the Error Reported broadcast VI is the only action performed by the \"Error\" message. The module's caller can then process the error appropriately."
              }
            }
            n113 = Merge Errors(w272, w271) -> (w267:errorcluster)
            n114 = local write "error out"(w267) -> ()
          }
          frame "Confirm Quit" {
            # "#CodeNeeded - If you want to provide an \"Are you sure\" dialog (or some other notification) before the application exits, place that code here. This message is typically sent from a Panel Close? event."
            # "Confirm Quit - Message that can confirm whether or not the user wants to exit the application."
            n115 = call-poly <vilib>:"Delacor_lib_QMH_Enqueue Message (poly).vi"("Priority Message? (F)"=TRUE, "error in"=w289, "Message"="Exit", "Message Queue in"=w285) -> ("error out"=w286:errorcluster)  [unwired: 6 in, 1 out]
            n116 = Merge Errors(w286) -> (w287:errorcluster)
          }
          frame "Exit" {
            w292 = FALSE ("Valve 1")
            w300 = 91  # 91: not all Exit messages will have an argument
            w305 = TRUE  # Stop the VI
            # "Release the message queue reference"
            # "Exit - Exit the application."
            n117 = Variant To Data(error in=w309, type=T10 {"Origin"="", "Exit via Stop Module Req?"=FALSE, "Wait for Module to stop?"=FALSE} ("Stop Argument"), Variant=w302) -> (data=w298:T10, error out=w301:errorcluster)
            n118 = call <vilib>:"Clear Errors.vi"("error in (no error)"=w301, "specific error code to clear (0: all)"=w300) -> ("error out"=w308:errorcluster)  [unwired: 4 in, 1 out]
            n119 = control-ref of="This VI"() -> (w296:refnum<vi>)
            n120 = call "Stop.vi"("Origin"="Ending Pressure Module") -> ()  [unwired: 10 in, 1 out]
            n121 = call "Stop.vi"("Origin"="Ending Actuator module") -> ()  [unwired: 10 in, 1 out]
            n122 = call-dynamic "Delacor_lib_QMH_Release Message Queue.vi"("error in"=w308, "Message Queue"=w307) -> ("error out"=w304:errorcluster)  [unwired: 9 in]
            n123 = call "Handle Exit.vi"("Stop Argument"=w298, "Admin in"=w295, "VI reference"=w296) -> ("error out"=w297:errorcluster)  [unwired: 7 in, 1 out]
            n124 = call "Stop.vi"("Origin"="Ending Temperature Module") -> ()  [unwired: 10 in, 1 out]
            n125 = call "Stop.vi"("Origin"="Ending Valve Module") -> ()  [unwired: 10 in, 1 out]
            n126 = local write "Valve 1"(w292) -> ()
            n127 = local write "Valve 2"(w292) -> ()
            n128 = local write "Valve 3"(w292) -> ()
            n129 = Merge Errors(w297, w304) -> (w303:errorcluster)
          }
          frame "Write Actuator" {
            # "Writing to actuator module"
            n130 = Variant To Data(error in=w316, type=0.0 ("NewVal"), Variant=w313) -> (data=w310:dbl, error out=w312:errorcluster)
            n131 = call "Set Actuator.vi"("Actuator"=w310) -> ()  [unwired: 10 in, 1 out]
            n132 = Merge Errors(w312) -> (w314:errorcluster)
          }
          frame Default {
            # "'Default' case only runs if there is a message that isn't defined in any of the other cases.  Output a programming error."
            n133 = call "Module Name--constant.vi"() -> ("Module Name"=w317:string)  [unwired: 11 in]
            n134 = xnode "Error Ring"("parameter 0"=w318, "parameter 1"=w317) -> ("error out"=w319:errorcluster)
          }
        }
        n135 = call-dynamic "Delacor_lib_QMH_Error Handler - Message Handling Loop.vi"("error in"=w176, "Message Queue in"=w167) -> ("dup error in"=w166:errorcluster)  [unwired: 8 in, 1 out]
      }
    }
    frame Error {
      # "Synchronize Caller Events.vi will inform Start Module.vi that the module has launched and will let the code calling Start Module.vi register for broadcasts and would permit the caller receive the broadcast that an error occurred at launch time."
      n136 = call "Synchronize Caller Events.vi"("Singleton Module Admin in"=w332) -> ("error out"=w329:errorcluster)  [unwired: 9 in, 1 out]
      n137 = call "Module Name--constant.vi"() -> ("Module Name"=w335:string)  [unwired: 11 in]
      n138 = Format Into String(format string="An error occurred during initialization. %s is no longer running.", w335) -> (resulting string=w333:string)  [unwired: 2 in, 1 out]
      n139 = Merge Errors(w331, w329) -> (w330:errorcluster)
      n140 = call "Error Reported.vi"("Additional Information"=w333, "Error"=w330) -> ()  [unwired: 9 in, 1 out]
    }
  }
  n141 = Merge Errors(w20, w28) -> (w14:errorcluster)
  n142 = call "Destroy Broadcast Events.vi"("error in (no error)"=w14) -> ("error out"=w11:errorcluster)  [unwired: 10 in]
  n143 = call "Destroy Broadcast Events.vi"("error in (no error)"=w11) -> ("error out"=w8:errorcluster)  [unwired: 10 in]
  n144 = call "Destroy Broadcast Events.vi"("error in (no error)"=w8) -> ("error out"=w2:errorcluster)  [unwired: 10 in]
  n145 = call "Destroy Broadcast Events.vi"("error in (no error)"=w2) -> ("error out"=w1:errorcluster)  [unwired: 10 in]
  n146 = call "Close Module.vi"("error in (no error)"=w1, "Module Admin in"=w29) -> ("error out"=w22:errorcluster, "External Launch"=w18:bool, "Module Admin out"=w21:refnum<class "Delacor_lib_QMH_Module Admin.lvclass">)  [unwired: 7 in]
  n147 = Unregister For Events(event registration refnum=w27, error in=w22) -> (error out=w19:errorcluster)
  "error out" <- w19
  n148 = local write "Module Admin"(w21) -> ()
  n149 = case "External Launch?" shown="True" w18 {
    tunnel: w19 -> [_ w337]
    frame False {
    }
    frame True {
      n150 = case shown="No Error" w337 {
        frame No Error {
          n151 = invoke class="VI" method="FP.Close"() -> ()  [unwired: 3 in, 3 out]
        }
        frame Error {
          n152 = invoke class="VI" method="FP.Open"("Activate"=TRUE ("Activate?")) -> ()  [unwired: 4 in, 5 out]
        }
      }
    }
  }
